vi "Test Copy Image to Pixmap With Mask ARGB.vi"(8 "error in (no error)":errorcluster, 11 "Test Case In":refnum<class "01_Image.lvclass">) -> (0 "error out":errorcluster, 3 "Test Case Out":refnum<class "01_Image.lvclass">)   [LabVIEW 2020, in "test.lvlib" / "01_Image.lvclass"]
uses:
  01_Image.lvclass
  C:/Program Files (x86)/National Instruments/LabVIEW 2026/vi.lib/Astemes/LUnit/Test Case.lvclass
  common/Image Size (Integer).ctl
  <vilib>/Astemes/LUnit/Test Case.lvclass/Test Case.ctl
  image/Match-Value Image (Colour).vi
  image/Copy Image to Pixmap (ARGB with Mask).vi
  4993e8ee-a06a-463a-9684-69129f64d5ce.vi
  image/New Image (Greyscale Preallocated).vi/6598b9e0-8a08-46f5-91fd-ca1b87217137.vi
  image/New Image.vi
  image/New Image (ARGB Preallocated).vi
  image/Copy Array to Image.vi
  image/Copy Array to Image (ARGB).vi
  image/Match-Value Image (Colour).vi/5701baee-35e2-4306-9a77-a9fdbb5b3a7f.vi
  image/Bitwise NOT (Greyscale).vi/f9ee80d6-438b-4cfb-91f1-04b98ac80474.vi
  image/Copy Image to Pixmap (ARGB with Mask).vi/5c639587-cf36-4d54-93d9-e654c7c24c6e.vi
  <vilib>/Astemes/LUnit/Core/LUnit Test Case/Private/Append Pass Result.vi
  <vilib>/Astemes/LUnit/Core/LUnit Test Case/Private/Append Fail Result.vi
  4993e8ee-a06a-463a-9684-69129f64d5ce.vi/9c5d11cd-9439-4240-a1ee-d9baace9c924.vi
  image/New Image (ARGB Preallocated).vi/3321fa97-f432-4e1e-8db9-a0df79aed21b.vi
  image/ARGB Colour to U32 Pixel Value.vi
  <vilib>/Astemes/LUnit/Core/LUnit Test Case/Private/Run In UI.vi
  <vilib>/Utility/error.llb/Clear Errors.vi
  <vilib>/Utility/error.llb/Error Cluster From Error Code.vi
  <vilib>/picture/pixmap.llb/Flatten Pixmap.vi
  common/common.lvlib
  image/image.lvlib
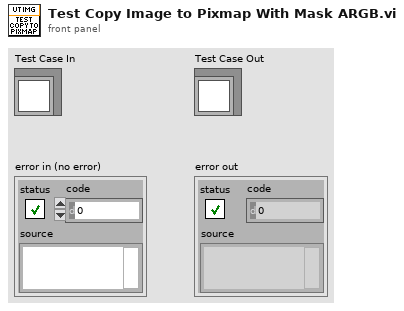
[diagram p1: front panel]
types:
  T1 = typedef "common.lvlib/Image Size (Integer).ctl" = cluster{"Width":u16, "Height":u16}
  T2 = typedef "image.lvlib/Greyscale Image.ctl" = refnum<data-value>
  T3 = typedef "image.lvlib/ARGB Image.ctl" = refnum<data-value>
  T4 = typedef "imagedata.ctl" = cluster{"image type":i32, "image depth":i32, "image":u8[], "mask":u8[], "colors":u32[], "Rectangle":cluster{"left":i16, "top":i16, "right":i16, "bottom":i16}}
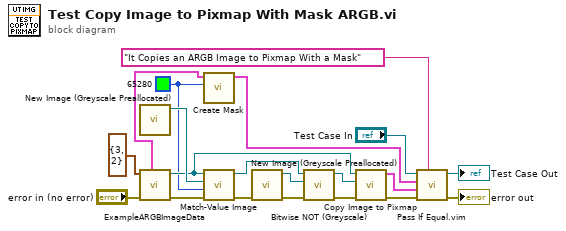
[diagram p0: block diagram]
diagram:
  w1 = u32 65280 ("RGB")
  n1 = call "New Image (Greyscale Preallocated).vi"() -> ("Greyscale Image"=w14:T2)  [unwired: 10 in, 1 out]
  n2 = call "ExampleARGBImageData.vi"("error in (no error)"="error in (no error)", "Image Size"=T1 {"Width"=3, "Height"=2} ("Preallocated Image Size (Default - 0,0)")) -> ("error out"=w12:errorcluster, "Data Value Reference out"=w13:T3, "ARGB Pixmap Data"=w15:T4)  [unwired: 6 in, 1 out]
  n3 = call <vilib>:"Create Mask.vi"("Mask Color (Black)"=w1, "image data"=w15) -> ("image data"=w5:T4)  [unwired: 9 in]
  n4 = call-poly "Match-Value Image.vi"("error in (no error)"=w12, "Value"=w1, "Match in"=w14, "ARGB Image Source in"=w13) -> ("error out"=w4:errorcluster, "Match Destination"=w8:T2)  [unwired: 6 in]
  n5 = call "New Image (Greyscale Preallocated).vi"("error in (no error)"=w4) -> ("error out"=w3:errorcluster, "Greyscale Image"=w7:T2)  [unwired: 9 in]
  n6 = call "Bitwise NOT (Greyscale).vi"("error in (no error)"=w3, "Greyscale Image Destination in"=w7, "Greyscale Image Source in"=w8) -> ("error out"=w9:errorcluster, "Greyscale Image Destination"=w2:T2)  [unwired: 7 in]
  n7 = call-poly "Copy Image to Pixmap.vi"("error in (no error)"=w9, "Greyscale Mask in"=w2, "ARGB Image Source in"=w13) -> ("error out"=w10:errorcluster, "Pixmap Image Data"=w6:T4)  [unwired: 7 in]
  n8 = call "Pass If Equal.vim"("Description"="It Copies an ARGB Image to Pixmap With a Mask", "error in (no error)"=w10, "Actual"=w6, "Expected"=w5, "LUnit Test Case In"="Test Case In") -> ("error out"=→"error out":errorcluster, "LUnit Test Case Out"=→"Test Case Out":refnum<class "01_Image.lvclass">)  [unwired: 5 in]
